vi "Generate Waveform.vi"(8 "error in (no error)":errorcluster, 11 "Simulated Waveform in":refnum<class "Simulated Waveform.lvclass">) -> (0 "error out":errorcluster, 3 "Simulated Waveform out":refnum<class "Simulated Waveform.lvclass">)   [LabVIEW 2020, in "Simulated Waveform.lvlib" / "Simulated Waveform.lvclass"]
uses:
  Simulated Waveform.lvclass
  Simulated Waveform.lvclass/Simulated Waveform.ctl
  build/ppl/Signal Generator.lvlibp/Signal Generator/Signal Generator.lvclass
  <vilib>/measure/NI_MABase.lvlib
  C:/dev/HAL Demo/build/ppl/Signal Generator.lvlibp/Signal Generator/Signal Generator.lvclass
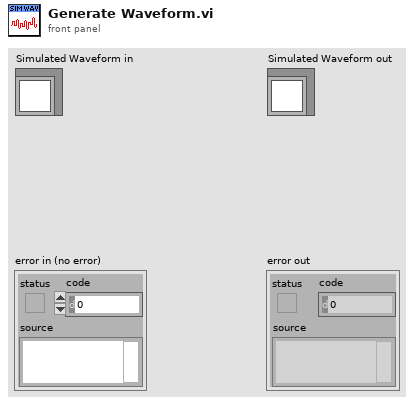
[diagram p1: front panel]
types:
  T1 = typedef "Signal Generator.lvlibp/Signal Generator.lvclass/Waveform Definition.ctl" = cluster{"Waveform Type":T2, "Frequency":dbl, "Amplitude":dbl}
  T2 = typedef "Signal Generator.lvlibp/Signal Generator.lvclass/Waveform Type.ctl" = enum16{"Sine Wave", "Triangle Wave", "Square Wave", "Sawtooth Wave"}
  T3 = typedef "Simulated Waveform.lvlib/Simulated Waveform.lvclass/Ref Data.ctl" = cluster{"Sim Queue Name":string, "Waveform Queue":refnum<queue>, "Noise Factor":dbl}
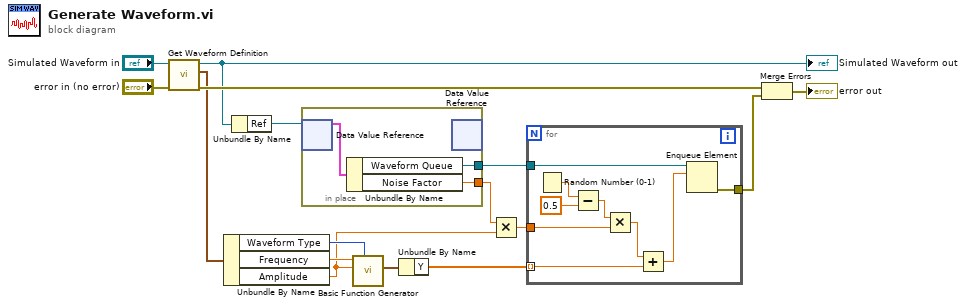
[diagram p0: block diagram]
diagram:
  n1 = call "Get Waveform Definition.vi"("error in (no error)"="error in (no error)", "Signal Generator in"="Simulated Waveform in") -> ("error out"=w13:errorcluster, "Waveform Definition"=w11:T1, "Signal Generator out"=w12:refnum<class "Simulated Waveform.lvclass">)  [unwired: 7 in]
  "Simulated Waveform out" <- w12
  n2 = Unbundle By Name(w11) -> ("Waveform Type"=w10:T2, "Frequency"=w9:dbl, "Amplitude"=w5:dbl)
  n3 = Unbundle By Name(w12) -> ("Ref"=w14:refnum<data-value>)
  n4 = in-place {
    in-place-border: [w18] -> w7
    in-place-border: [w17] -> w4
    n5 = in-place-dvr #1(w14) -> (w19:T3)  [unwired: 1 out]
    n6 = Unbundle By Name(w19) -> ("Waveform Queue"=w18:refnum<queue>, "Noise Factor"=w17:dbl)
    n7 = in-place-dvr #1() -> ()  [unwired: 1 in, 2 out]
  }
  n8 = call <vilib>:"Basic Function Generator.vi"("signal type"=w10, "amplitude"=w5, "frequency"=w9) -> ("signal out"=w8:waveform(dbl))  [unwired: 6 in, 2 out]
  n9 = Unbundle By Name(w8) -> ("Y"=w6:dbl[])
  n10 = Multiply(x=w4, y=w5) -> (x*y=w3:dbl)
  n11 = for {
    tunnel: w7 -> [w28]
    tunnel: w6 -> [w23] mode=indexing
    tunnel: w3 -> [w25]
    tunnel: [w20] -> w1
    n12 = Random Number (0-1)() -> (number: 0 to 1=w27:dbl)
    n13 = Subtract(x=w27, y=0.5) -> (x-y=w24:dbl)
    n14 = Multiply(x=w24, y=w25) -> (x*y=w22:dbl)
    n15 = Add(x=w22, y=w23) -> (x+y=w21:dbl)
    n16 = Enqueue Element(queue=w28, element=w21) -> (error out=w20:errorcluster)  [unwired: 2 in, 2 out]
  }
  n17 = Merge Errors(w13, w1) -> (→"error out":errorcluster)
